vi "Creator Queue.vi"(9 "Priority?":bool, 10 "Msg Strategy":refnum<class "Msg Strategy.lvclass">, 11 "Base Queue in":refnum<class "Base Queue.lvclass">) -> (3 "Base Queue out":refnum<class "Base Queue.lvclass">)   [LabVIEW 2021, in "jettl.lvlib" / "Base Queue.lvlib" / "Base Queue.lvclass"]
uses:
  Base Queue.lvclass
  C:/git/jettl/src/jettl/jettl/jettl.lvclass
  Msg Strategy/Msg Strategy.lvclass
  Base Queue.lvclass/Base Queue.ctl
  Queue Mailbox/Queue Mailbox.lvlib
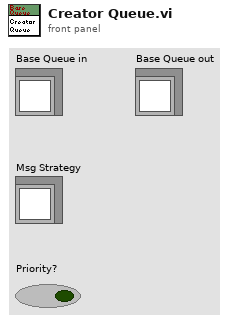
[diagram p1: front panel]
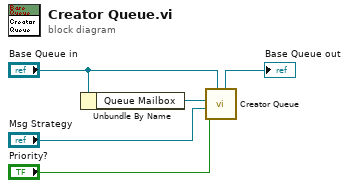
[diagram p0: block diagram]
diagram:
  n1 = Unbundle By Name("Base Queue in") -> ("Queue Mailbox"=w5:refnum<data-value>)
  n2 = call "Creator Queue.vi"("jettl in"="Base Queue in", "Priority?"="Priority?", "Msg Strategy"="Msg Strategy", "Queue Mailbox"=w5) -> ("jettl out"=→"Base Queue out":refnum<class "Base Queue.lvclass">)  [unwired: 7 in]
